vi "VeriStand Framework Configuration.Set Device Reference.vi"(10 "Device Item Ref":T1=18446744073709551615 format="%.0x", 11 "VeriStand Framework Configuration in":refnum<class "VeriStand DSF.Framework.Configuration.lvclass">=refnum) -> (3 "VeriStand Framework Configuration out":refnum<class "VeriStand DSF.Framework.Configuration.lvclass">)   [LabVIEW 2017, in "Data Sharing Custom Device Engine.lvlib" / "VeriStand DSF.Framework.Configuration.lvclass"]
uses:
  VeriStand DSF.Framework.Configuration.lvclass
  <vilib>/NI Veristand/Custom Device API/Custom Device Item Ref.ctl
  VeriStand DSF.Framework.Configuration.lvclass/VeriStand DSF.Framework.Configuration.ctl
  <vilib>/NI Veristand/Custom Device API/Custom Device API.lvlib
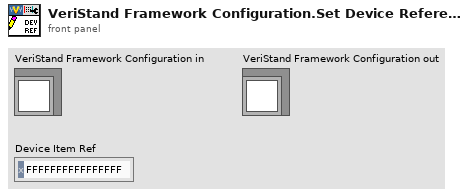
[diagram p1: front panel]
types:
  T1 = typedef "Custom Device API.lvlib/Custom Device Item Ref.ctl" = u64
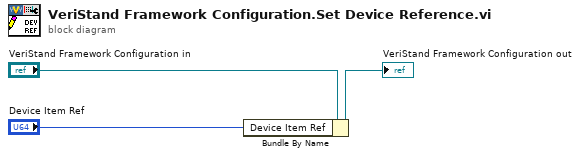
[diagram p0: block diagram]
diagram:
  n1 = Bundle By Name(cluster="VeriStand Framework Configuration in", "Device Item Ref"="Device Item Ref") -> (→"VeriStand Framework Configuration out":refnum<class "VeriStand DSF.Framework.Configuration.lvclass">)
